vi "PDF Protokoll CalGas.vi"(8 "error in (no error)":errorcluster caption="Fehler (Eingang, kein Fehler)", 11 "Zeitstempel":timestamp) -> (0 "error out":errorcluster caption="Fehler (Ausgang)")   [LabVIEW 2020, in "Erweiterte Konfig.lvlib" / "CG-Check Konfig.lvlib"]
uses:
  CG-Check Konfig.lvlib
  Sprachverwaltung/FGV Aktion Tabelle zerlegen.ctl
  System Einstellungen V2/Aktioen FGV System Konstanten.ctl
  Aktion_CG-Check.ctl
  Schedule Modul/Aktion FGV Testdaten sammeln.ctl
  FT-IR/FGV FT-IR Gasliste Aktionen.ctl
  Gaszuordnung AO/FGV Gaszuordnung Grenzen&Einheit Aktion.ctl
  <vilib>/Utility/miscctls.llb/LVPrintingMarginsTypeDef.ctl
  Schedule Modul/Schedule Modul.lvlib
  System Einstellungen V2/System Einstellungen V2.lvlib
  FT-IR/FT-IR.lvlib
  Gaszuordnung AO/Gaszuordnung AO.lvlib
  Allgemein/allgemeine Sub-VIs.lvlib
  Sprachverwaltung/Sprachverwaltung.lvlib
panel:
  out "Span Eingang 3":string[][](table) caption="Span Inlet 3"
  out "Ergebnis 3":string caption="Result:"
  out "Span Eingang 2":string[][](table) caption="Span Inlet 2"
  out "Ergebnis 2":string caption="Result:"
  out "Span Eingang 1":string[][](table) caption="Span Inlet 1"
  out "Ergebnis":string caption="Result:"
  out "Datum":string caption="Date:"
  out "Messgerät:":string caption="Analyzer:"
  # "Calibration Gas Test Protocol"
  # "Results:"
  # "IAG-Industrie Automatisierungsgeschellschaft m.b.H.    l  Industriestraße 322    l    2722Weikersdorf     )+43262241712/0"
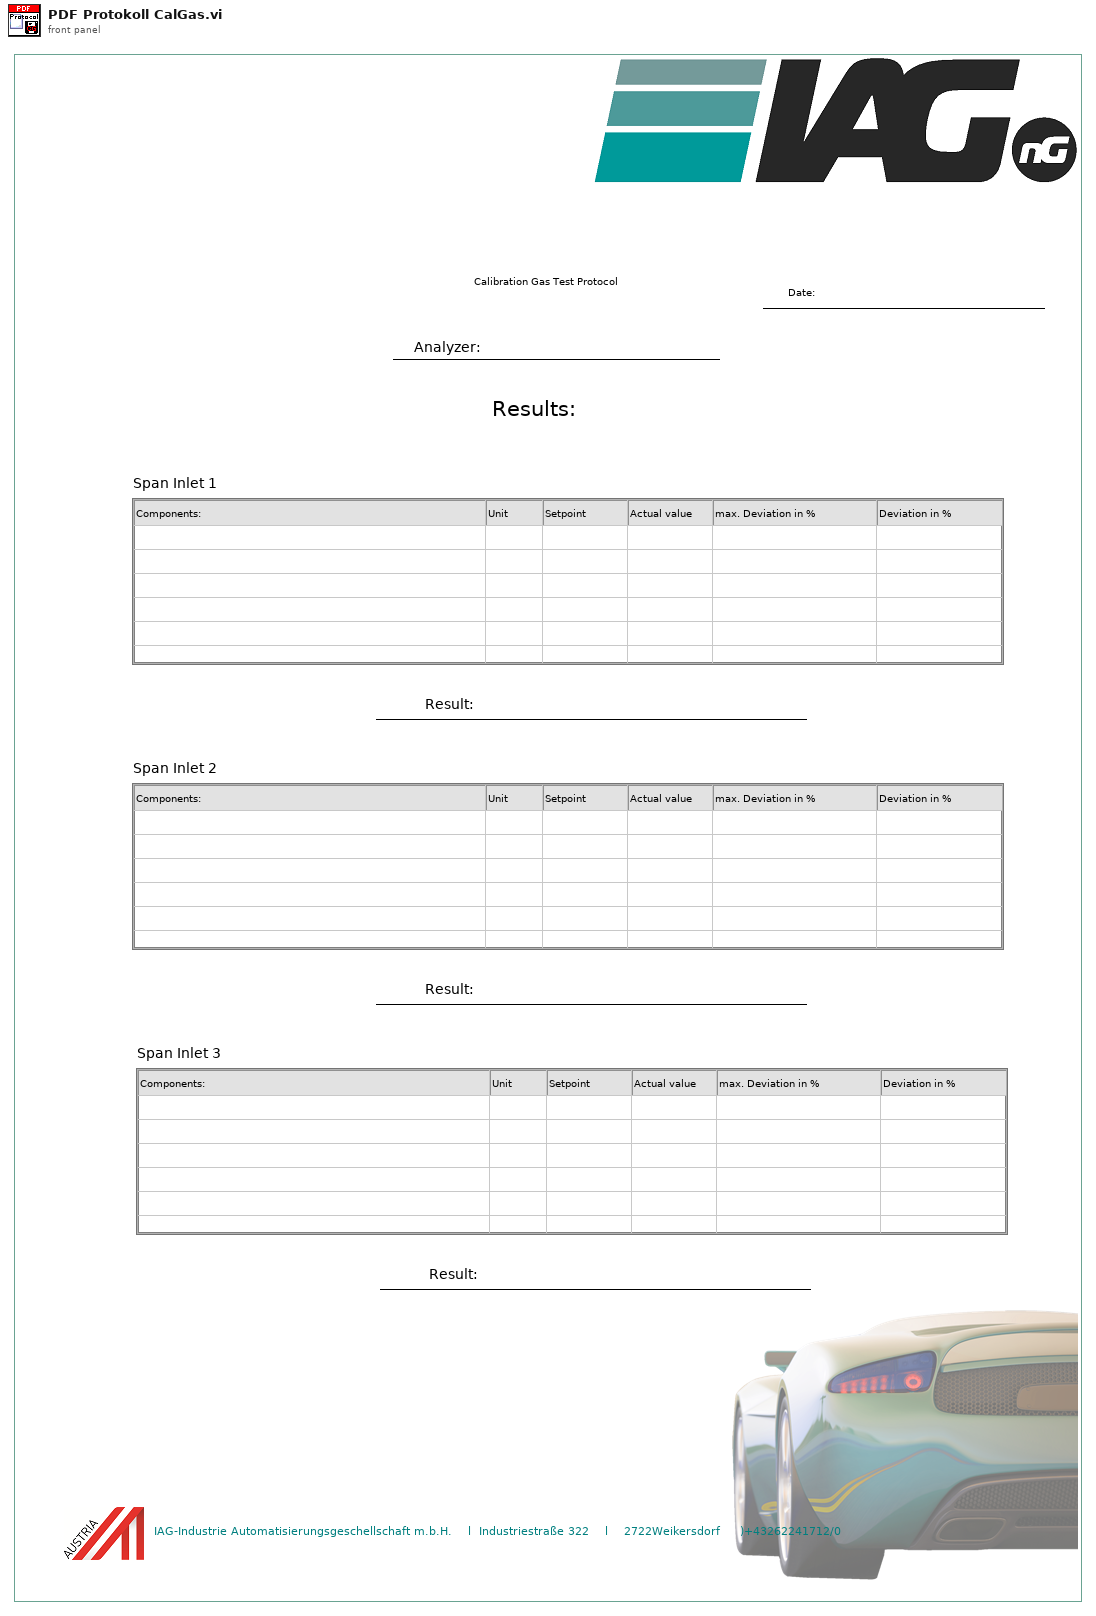
[diagram p1: front panel]
types:
  T1 = typedef "Sprachverwaltung.lvlib/FGV Aktion Tabelle zerlegen.ctl" = enum16{"laden", "vereinzeln", "speichern"}
  T2 = typedef "Schedule Modul.lvlib/Aktion FGV Testdaten sammeln.ctl" = enum16{"lesen", "Dichtheitstest", "CalGasTest", "T90", "Kalibrieren", "init", "Kalender Daten"}
  T3 = typedef "Erweiterte Konfig.lvlib/CG-Check Konfig.lvlib/Aktion_CG-Check.ctl" = enum16{"lesen", "schreiben", "laden", "Komponente", "Aktive?", "speichern"}
  T4 = typedef "System Einstellungen V2.lvlib/Aktioen FGV System Konstanten.ctl" = enum16{"lesen", "laden", "speichern", "Sprache"}
  T5 = typedef "FT-IR.lvlib/FGV FT-IR Gasliste Aktionen.ctl" = enum16{"lesen", "Gasliste FT-IR", "Gasliste ausgelesen", "laden", "speichern", "löschen"}
  T6 = typedef "Gaszuordnung AO.lvlib/FGV Gaszuordnung Grenzen&Einheit Aktion.ctl" = enum16{"Lesen", "Schreiben Min", "Schreiben Max", "Laden", "Speichern"}
  T7 = enum32{"Portrait", "Landscape", "Rotated Portrait", "Rotated Landscape"}
  T8 = typedef "LVPrintingMarginsTypeDef.ctl" = cluster{"Top":sgl, "Left":sgl, "Bottom":sgl, "Right":sgl, "Measurement System":enum8{"Inches", "cm"}}
  T9 = typedef "Schedule Modul.lvlib/Ergebnis CalGas Test.ctl" = cluster{"Istwerte":string[][], "Auswertung":string[][][], "Fehler":bool[], "Abweichung in %":string[][], "Spanauswahl":i32[]}
  T10 = typedef "String - Ausgabefeld.ctl" = string
  T11 = cluster{"Modell":string, "ProjektNummer":string, "Software Version":string, "Seriennummer":string}
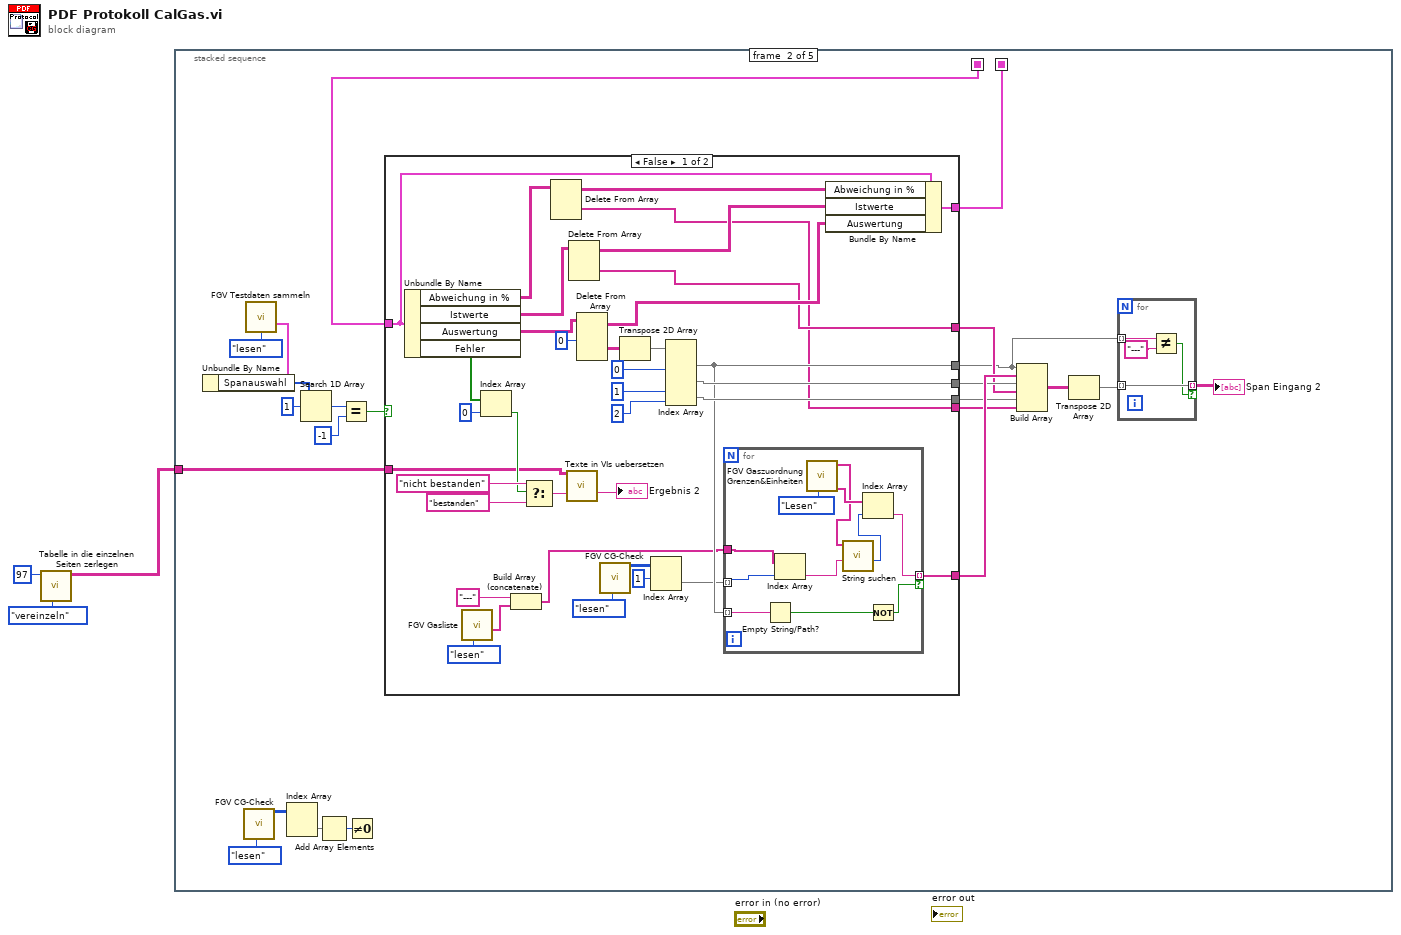
[diagram p0: block diagram]
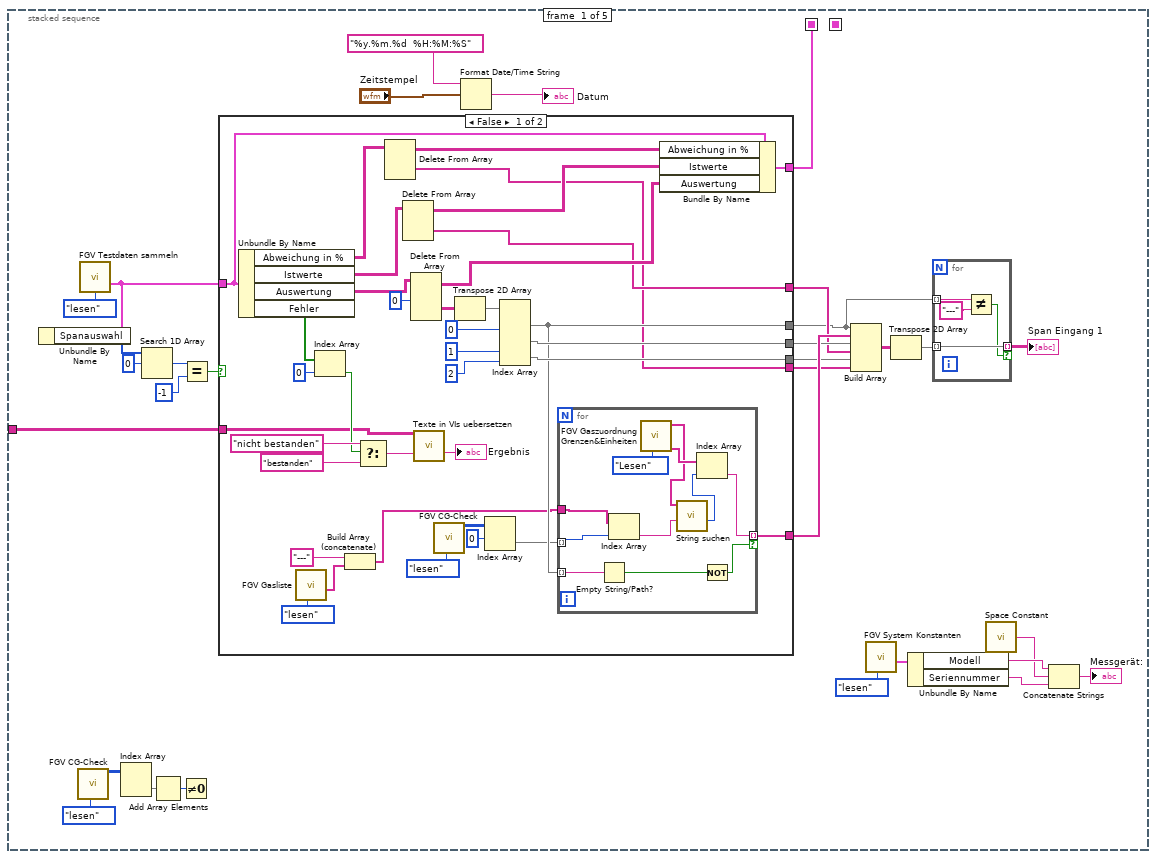
[diagram p2: hidden frame]
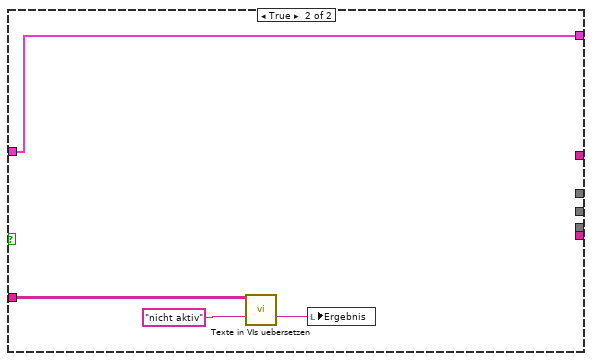
[diagram p3: hidden frame]
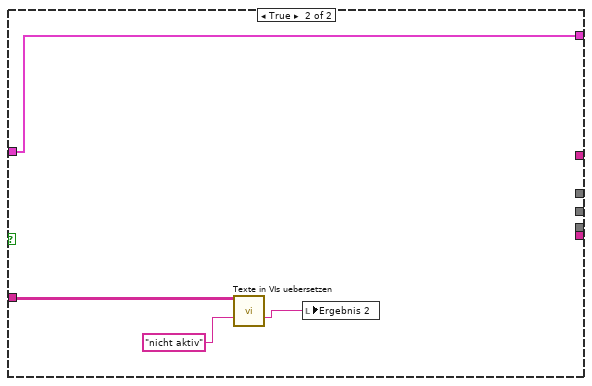
[diagram p4: hidden frame]
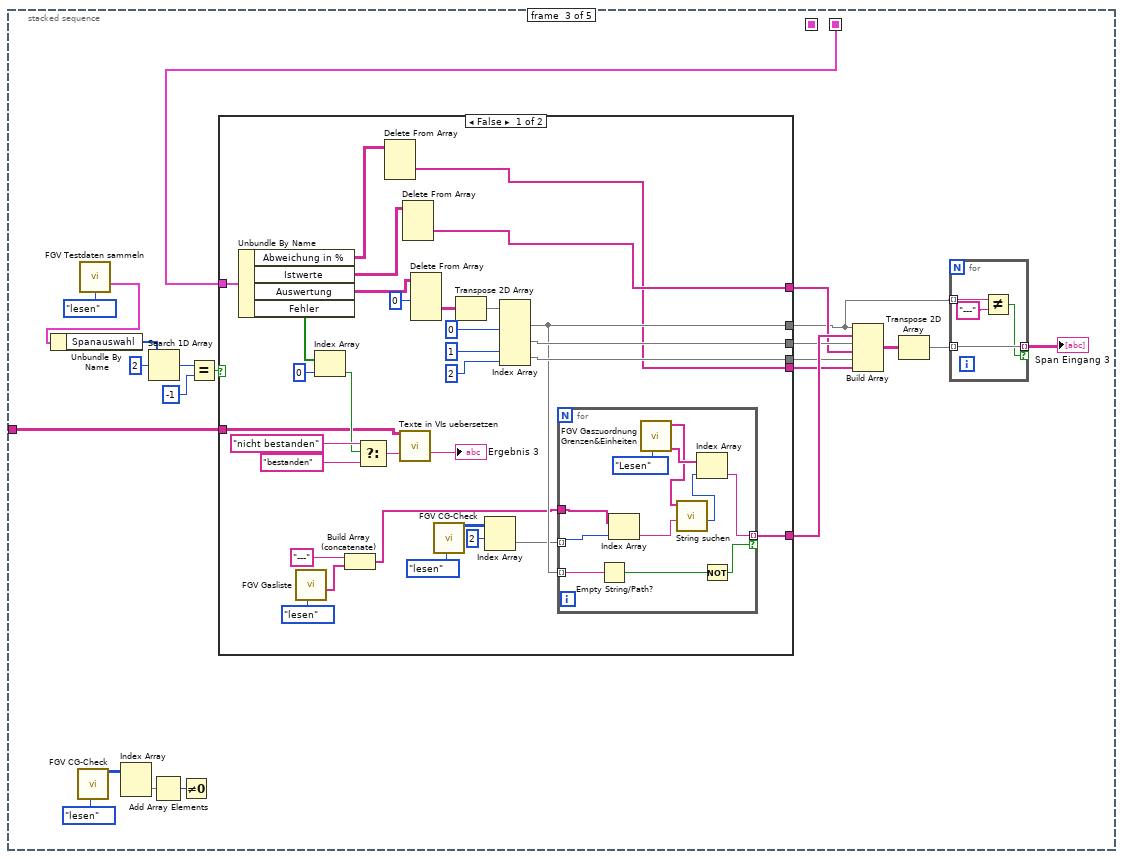
[diagram p5: hidden frame]
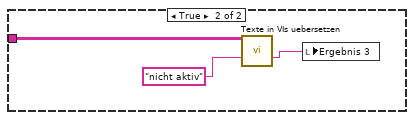
[diagram p6: hidden frame]
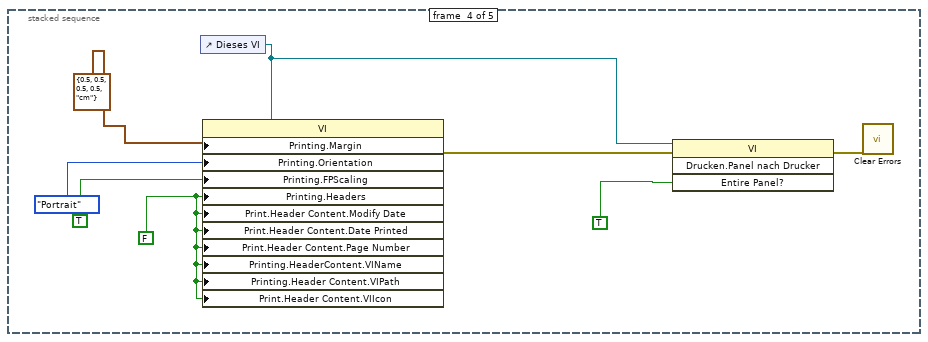
[diagram p7: hidden frame]
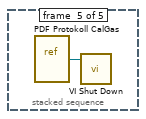
[diagram p8: hidden frame]
diagram:
  n1 = call "Tabelle in die einzelnen Seiten zerlegen.vi"("Aktion"=FGV_Aktion_Tabelle_zerlegen."vereinzeln", "Index (Seite)"=97) -> ("Sprachliste"=w1:string[][])  [unwired: 7 in, 2 out]
  n2 = stacked-sequence {
    seq-local: [w13 _ _ _ _] -> [_ w100 _ _ _]
    seq-local: [_ w99 _ _ _] -> [_ _ w179 _ _]
    tunnel: w1 -> [w4 w90 w168 _ _]
    frame #0 {
      n3 = call "FGV CG-Check.vi"("Aktion"=Aktion_CG-Check."lesen") -> ("Komponenten"=w17:u16[][])  [unwired: 11 in, 7 out]
      n4 = call "FGV Testdaten sammeln.vi"("Aktion"=Aktion_FGV_Testdaten_sammeln."lesen") -> ("Ergebnis CalGas Test"=w15:T9)  [unwired: 9 in, 5 out]
      n5 = Unbundle By Name(w15) -> ("Spanauswahl"=w12:i32[])
      n6 = Index Array(array=w17) -> (element=w19:u16[])  [unwired: 2 in]
      n7 = Search 1D Array(1D array=w12, element=0 ("Element")) -> (index of element=w10:i32)  [unwired: 1 in]
      n8 = Add Array Elements(numeric array=w19) -> (sum=w20:u16)
      n9 = Not Equal To 0?(x=w20) -> ()  [unwired: 1 out]
      n10 = Equal?(x=w10, y=-1) -> (x = y?=w14:bool)
      n11 = case shown="False" w14 {
        tunnel: [w61 _] -> w5
        tunnel: [w60 _] -> w25
        tunnel: [w71 _] -> w24
        tunnel: [w46 _] -> w23
        tunnel: [w70 _] -> w22
        tunnel: [w45 _] -> w21
        tunnel: w15 -> [w53 w89]
        tunnel: [w44 w89] -> w13
        tunnel: w4 -> [w39 w86]
        frame False {
          n12 = Unbundle By Name(w53) -> ("Abweichung in %"=w69:string[][], "Istwerte"=w51:string[][], "Auswertung"=w49:string[][][], "Fehler"=w66:bool[])
          n13 = call "FGV Gasliste.vi"("Aktionen"=FGV_FT-IR_Gasliste_Aktionen."lesen") -> ("Aktuelle Gasliste gesamt"=w56:T10[])  [unwired: 8 in, 2 out]
          n14 = Index Array(array=w66, index=0 ("Index")) -> (element=w64:bool)
          n15 = Build Array (concatenate)("---", w56) -> (w55:T10[])
          n16 = Select(t="nicht bestanden" ("String"), s=w64, f="bestanden" ("String")) -> (s? t:f=w41:string)
          n17 = Delete From Array(array=w69) -> (deleted portion=w45:string[], array with subset deleted=w52:string[][])  [unwired: 3 in]
          n18 = Delete From Array(array=w51) -> (deleted portion=w46:string[], array with subset deleted=w50:string[][])  [unwired: 3 in]
          n19 = Delete From Array(array=w49, index (dim 0)=0 ("Index (Seite)")) -> (deleted portion=w47:string[][], array with subset deleted=w48:string[][][])  [unwired: 3 in]
          n20 = call "Texte in VIs uebersetzen.vi"("Sprachliste"=w39, "String zum Übersetzen"=w41) -> ("String zum Übersetzen"=→"Ergebnis":string)  [unwired: 9 in, 4 out]
          n21 = call "FGV CG-Check.vi"("Aktion"=Aktion_CG-Check."lesen") -> ("Komponenten"=w62:u16[][])  [unwired: 11 in, 7 out]
          n22 = Transpose 2D Array(2D array=w47) -> (transposed array=w42:string[][])
          n23 = Index Array(array=w62, index (row)=0 ("Index (Zeile)")) -> (element=w54:u16[])  [unwired: 1 in]
          n24 = Index Array(array=w42, index (col) #1=0 ("Deaktivierter Index (Zeile)"), index (col) #2=1 ("Deaktivierter Index (Zeile)"), index (col) #3=2 ("Deaktivierter Index (Zeile)")) -> (element #1=w61:string[], element #2=w71:string[], element #3=w70:string[])  [unwired: 3 in]
          n25 = for {
            tunnel: w61 -> [w80] mode=indexing
            tunnel: [w83] -> w60 mode=indexing if=w81
            tunnel: w55 -> [w79]
            tunnel: w54 -> [w78] mode=indexing
            n26 = Empty String/Path?(string/path=w80) -> (empty?=w82:bool)
            n27 = Index Array(array=w79, index=w78) -> (element=w76:T10)
            n28 = call "FGV Gaszuordnung Grenzen&Einheiten.vi"("Aktion"=FGV_Gaszuordnung_Grenzen&Einheit_Aktion."Lesen") -> ("Einheit neu"=w84:string[], "Namen neu"=w77:string[])  [unwired: 7 in, 2 out]
            n29 = call "String suchen.vi"("Gasname"=w76, "Such-Namen"=w77) -> ("Index"=w75:i32)  [unwired: 8 in, 1 out]
            n30 = Index Array(array=w84, index=w75) -> (element=w83:string)
            n31 = Not(x=w82) -> (.not. x?=w81:bool)
          }
          n32 = Bundle By Name(cluster=w53, "Abweichung in %"=w52, "Istwerte"=w50, "Auswertung"=w48) -> (w44:T9)
        }
        frame True {
          n33 = call "Texte in VIs uebersetzen.vi"("Sprachliste"=w86, "String zum Übersetzen"="nicht aktiv" ("f")) -> ("String zum Übersetzen"=w87:string)  [unwired: 9 in, 4 out]
          n34 = local write "Ergebnis"(w87) -> ()
        }
      }
      n35 = Format Date/Time String(time format string (%c)="%y.%m.%d  %H:%M:%S" ("Zeitformatierungs-String (%c)"), seconds (now)="Zeitstempel") -> (date/time string=→"Datum":string)  [unwired: 1 in]
      n36 = Build Array(w5, w25, w24, w23, w22, w21) -> (w8:string[][])
      n37 = call "FGV System Konstanten.vi"("Aktionen"=Aktioen_FGV_System_Konstanten."lesen") -> ("Cluster out"=w33:T11)  [unwired: 6 in, 4 out]
      n38 = Transpose 2D Array(2D array=w8) -> (transposed array=w7:string[][])
      n39 = Unbundle By Name(w33) -> ("Modell"=w32:string, "Seriennummer"=w30:string)
      n40 = for {
        tunnel: [w38] -> w6 mode=indexing if=w35
        tunnel: w7 -> [w38] mode=indexing
        tunnel: w5 -> [w37] mode=indexing
        n41 = Not Equal?(x=w37, y="---") -> (x != y?=w35:bool)
      }
      "Span Eingang 1" <- w6
      n42 = call <vilib>:"Space Constant.vi"() -> ("String"=w31:string)
      n43 = Concatenate Strings(w32, w31, w30) -> (→"Messgerät:":string)
    }
    frame #1 {
      n44 = call "FGV CG-Check.vi"("Aktion"=Aktion_CG-Check."lesen") -> ("Komponenten"=w104:u16[][])  [unwired: 11 in, 7 out]
      n45 = call "FGV Testdaten sammeln.vi"("Aktion"=Aktion_FGV_Testdaten_sammeln."lesen") -> ("Ergebnis CalGas Test"=w102:T9)  [unwired: 9 in, 5 out]
      n46 = Unbundle By Name(w102) -> ("Spanauswahl"=w97:i32[])
      n47 = Index Array(array=w104) -> (element=w106:u16[])  [unwired: 2 in]
      n48 = Search 1D Array(1D array=w97, element=1 ("Element")) -> (index of element=w96:i32)  [unwired: 1 in]
      n49 = Add Array Elements(numeric array=w106) -> (sum=w107:u16)
      n50 = Equal?(x=w96, y=-1) -> (x = y?=w101:bool)
      n51 = Not Equal To 0?(x=w107) -> ()  [unwired: 1 out]
      n52 = case shown="False" w101 {
        tunnel: [w139 _] -> w91
        tunnel: [w138 _] -> w112
        tunnel: [w149 _] -> w111
        tunnel: [w124 _] -> w110
        tunnel: [w148 _] -> w109
        tunnel: [w123 _] -> w108
        tunnel: w100 -> [w131 w167]
        tunnel: [w122 w167] -> w99
        tunnel: w90 -> [w117 w164]
        frame False {
          n53 = Unbundle By Name(w131) -> ("Abweichung in %"=w147:string[][], "Istwerte"=w129:string[][], "Auswertung"=w127:string[][][], "Fehler"=w144:bool[])
          n54 = call "FGV Gasliste.vi"("Aktionen"=FGV_FT-IR_Gasliste_Aktionen."lesen") -> ("Aktuelle Gasliste gesamt"=w134:T10[])  [unwired: 8 in, 2 out]
          n55 = Index Array(array=w144, index=0 ("Index")) -> (element=w142:bool)
          n56 = Build Array (concatenate)("---", w134) -> (w133:T10[])
          n57 = Select(t="nicht bestanden" ("String"), s=w142, f="bestanden" ("String")) -> (s? t:f=w119:string)
          n58 = Delete From Array(array=w147) -> (deleted portion=w123:string[], array with subset deleted=w130:string[][])  [unwired: 3 in]
          n59 = call "Texte in VIs uebersetzen.vi"("Sprachliste"=w117, "String zum Übersetzen"=w119) -> ("String zum Übersetzen"=→"Ergebnis 2":string)  [unwired: 9 in, 4 out]
          n60 = Delete From Array(array=w129) -> (deleted portion=w124:string[], array with subset deleted=w128:string[][])  [unwired: 3 in]
          n61 = Delete From Array(array=w127, index (dim 0)=0 ("Index (Seite)")) -> (deleted portion=w125:string[][], array with subset deleted=w126:string[][][])  [unwired: 3 in]
          n62 = call "FGV CG-Check.vi"("Aktion"=Aktion_CG-Check."lesen") -> ("Komponenten"=w140:u16[][])  [unwired: 11 in, 7 out]
          n63 = Transpose 2D Array(2D array=w125) -> (transposed array=w120:string[][])
          n64 = Index Array(array=w140, index (row)=1 ("Index (Zeile)")) -> (element=w132:u16[])  [unwired: 1 in]
          n65 = Index Array(array=w120, index (col) #1=0 ("Deaktivierter Index (Zeile)"), index (col) #2=1 ("Deaktivierter Index (Zeile)"), index (col) #3=2 ("Deaktivierter Index (Zeile)")) -> (element #1=w139:string[], element #2=w149:string[], element #3=w148:string[])  [unwired: 3 in]
          n66 = for {
            tunnel: w139 -> [w158] mode=indexing
            tunnel: [w161] -> w138 mode=indexing if=w159
            tunnel: w133 -> [w157]
            tunnel: w132 -> [w156] mode=indexing
            n67 = Empty String/Path?(string/path=w158) -> (empty?=w160:bool)
            n68 = Index Array(array=w157, index=w156) -> (element=w154:T10)
            n69 = call "FGV Gaszuordnung Grenzen&Einheiten.vi"("Aktion"=FGV_Gaszuordnung_Grenzen&Einheit_Aktion."Lesen") -> ("Einheit neu"=w162:string[], "Namen neu"=w155:string[])  [unwired: 7 in, 2 out]
            n70 = call "String suchen.vi"("Gasname"=w154, "Such-Namen"=w155) -> ("Index"=w153:i32)  [unwired: 8 in, 1 out]
            n71 = Index Array(array=w162, index=w153) -> (element=w161:string)
            n72 = Not(x=w160) -> (.not. x?=w159:bool)
          }
          n73 = Bundle By Name(cluster=w131, "Abweichung in %"=w130, "Istwerte"=w128, "Auswertung"=w126) -> (w122:T9)
        }
        frame True {
          n74 = call "Texte in VIs uebersetzen.vi"("Sprachliste"=w164, "String zum Übersetzen"="nicht aktiv" ("f")) -> ("String zum Übersetzen"=w165:string)  [unwired: 9 in, 4 out]
          n75 = local write "Ergebnis 2"(w165) -> ()
        }
      }
      n76 = Build Array(w91, w112, w111, w110, w109, w108) -> (w94:string[][])
      n77 = Transpose 2D Array(2D array=w94) -> (transposed array=w93:string[][])
      n78 = for {
        tunnel: [w116] -> w92 mode=indexing if=w113
        tunnel: w93 -> [w116] mode=indexing
        tunnel: w91 -> [w115] mode=indexing
        n79 = Not Equal?(x=w115, y="---") -> (x != y?=w113:bool)
      }
      "Span Eingang 2" <- w92
    }
    frame #2 {
      n80 = call "FGV CG-Check.vi"("Aktion"=Aktion_CG-Check."lesen") -> ("Komponenten"=w181:u16[][])  [unwired: 11 in, 7 out]
      n81 = call "FGV Testdaten sammeln.vi"("Aktion"=Aktion_FGV_Testdaten_sammeln."lesen") -> ("Ergebnis CalGas Test"=w174:T9)  [unwired: 9 in, 5 out]
      n82 = Unbundle By Name(w174) -> ("Spanauswahl"=w175:i32[])
      n83 = Index Array(array=w181) -> (element=w183:u16[])  [unwired: 2 in]
      n84 = Search 1D Array(1D array=w175, element=2 ("Element")) -> (index of element=w177:i32)  [unwired: 1 in]
      n85 = Add Array Elements(numeric array=w183) -> (sum=w184:u16)
      n86 = Not Equal To 0?(x=w184) -> ()  [unwired: 1 out]
      n87 = Equal?(x=w177, y=-1) -> (x = y?=w173:bool)
      n88 = case shown="False" w173 {
        tunnel: [w212 _] -> w169
        tunnel: [w211 _] -> w189
        tunnel: [w222 _] -> w188
        tunnel: [w200 _] -> w187
        tunnel: [w221 _] -> w186
        tunnel: [w199 _] -> w185
        tunnel: w179 -> [w204 _]
        tunnel: w168 -> [w194 w237]
        frame False {
          n89 = Unbundle By Name(w204) -> ("Abweichung in %"=w220:string[][], "Istwerte"=w203:string[][], "Auswertung"=w202:string[][][], "Fehler"=w217:bool[])
          n90 = call "FGV Gasliste.vi"("Aktionen"=FGV_FT-IR_Gasliste_Aktionen."lesen") -> ("Aktuelle Gasliste gesamt"=w207:T10[])  [unwired: 8 in, 2 out]
          n91 = Index Array(array=w217, index=0 ("Index")) -> (element=w215:bool)
          n92 = Build Array (concatenate)("---", w207) -> (w206:T10[])
          n93 = Select(t="nicht bestanden" ("String"), s=w215, f="bestanden" ("String")) -> (s? t:f=w196:string)
          n94 = Delete From Array(array=w220) -> (deleted portion=w199:string[])  [unwired: 3 in, 1 out]
          n95 = call "Texte in VIs uebersetzen.vi"("Sprachliste"=w194, "String zum Übersetzen"=w196) -> ("String zum Übersetzen"=→"Ergebnis 3":string)  [unwired: 9 in, 4 out]
          n96 = Delete From Array(array=w203) -> (deleted portion=w200:string[])  [unwired: 3 in, 1 out]
          n97 = Delete From Array(array=w202, index (dim 0)=0 ("Index (Seite)")) -> (deleted portion=w201:string[][])  [unwired: 3 in, 1 out]
          n98 = call "FGV CG-Check.vi"("Aktion"=Aktion_CG-Check."lesen") -> ("Komponenten"=w213:u16[][])  [unwired: 11 in, 7 out]
          n99 = Transpose 2D Array(2D array=w201) -> (transposed array=w197:string[][])
          n100 = Index Array(array=w213, index (row)=2 ("Index (Zeile)")) -> (element=w205:u16[])  [unwired: 1 in]
          n101 = Index Array(array=w197, index (col) #1=0 ("Deaktivierter Index (Zeile)"), index (col) #2=1 ("Deaktivierter Index (Zeile)"), index (col) #3=2 ("Deaktivierter Index (Zeile)")) -> (element #1=w212:string[], element #2=w222:string[], element #3=w221:string[])  [unwired: 3 in]
          n102 = for {
            tunnel: w212 -> [w231] mode=indexing
            tunnel: [w234] -> w211 mode=indexing if=w232
            tunnel: w206 -> [w230]
            tunnel: w205 -> [w229] mode=indexing
            n103 = Empty String/Path?(string/path=w231) -> (empty?=w233:bool)
            n104 = Index Array(array=w230, index=w229) -> (element=w227:T10)
            n105 = call "FGV Gaszuordnung Grenzen&Einheiten.vi"("Aktion"=FGV_Gaszuordnung_Grenzen&Einheit_Aktion."Lesen") -> ("Einheit neu"=w235:string[], "Namen neu"=w228:string[])  [unwired: 7 in, 2 out]
            n106 = call "String suchen.vi"("Gasname"=w227, "Such-Namen"=w228) -> ("Index"=w226:i32)  [unwired: 8 in, 1 out]
            n107 = Index Array(array=w235, index=w226) -> (element=w234:string)
            n108 = Not(x=w233) -> (.not. x?=w232:bool)
          }
        }
        frame True {
          n109 = call "Texte in VIs uebersetzen.vi"("Sprachliste"=w237, "String zum Übersetzen"="nicht aktiv" ("f")) -> ("String zum Übersetzen"=w239:string)  [unwired: 9 in, 4 out]
          n110 = local write "Ergebnis 3"(w239) -> ()
        }
      }
      n111 = Build Array(w169, w189, w188, w187, w186, w185) -> (w172:string[][])
      n112 = Transpose 2D Array(2D array=w172) -> (transposed array=w171:string[][])
      n113 = for {
        tunnel: [w193] -> w170 mode=indexing if=w190
        tunnel: w171 -> [w193] mode=indexing
        tunnel: w169 -> [w192] mode=indexing
        n114 = Not Equal?(x=w192, y="---") -> (x != y?=w190:bool)
      }
      "Span Eingang 3" <- w170
    }
    frame #3 {
      w243 = FALSE ("Drucken:Kopfzeilen?")
      n115 = control-ref of="Dieses VI"() -> (w240:refnum<vi>)
      n116 = property class="VI"(reference=w240, "Printing.Margin"=T8 {"Top"=0.5, "Left"=0.5, "Bottom"=0.5, "Right"=0.5, "Measurement System"=enum."cm"} ("Drucken:Ränder"), "Printing.Orientation"=T7."Portrait" ("Drucken:Seitenausrichtung"), "Printing.FPScaling"=TRUE ("Drucken:Frontpanel-Skalierung?"), "Printing.Headers"=w243, "Print.Header Content.Modify Date"=w243, "Print.Header Content.Date Printed"=w243, "Print.Header Content.Page Number"=w243, "Printing.HeaderContent.VIName"=w243, "Printing.Header Content.VIPath"=w243, "Print.Header Content.VIIcon"=w243) -> (error out=w247:errorcluster)  [unwired: 1 in, 1 out]
      n117 = invoke class="VI" method="Drucken.Panel nach Drucker"(reference=w240, error in=w247, "Entire Panel?"=TRUE ("Abschnittskopfzeilen?")) -> (error out=w241:errorcluster)  [unwired: 1 in, 3 out]
      n118 = call <vilib>:"Clear Errors.vi"("error in (no error)"=w241) -> ()  [unwired: 5 in, 2 out]
    }
    frame #4 {
      n119 = vi-ref "PDF Protokoll CalGas.vi"() -> (w248:refnum<vi>)
      n120 = call "VI Shut Down.vi"("VI Referenz"=w248) -> ()  [unwired: 11 in]
    }
  }
